vi "LogicEditor.vi"(1 "Logic Express":string) -> (0 "LogicExpressOut":string)   [LabVIEW 2020]
uses:
  <vilib>/Utility/miscctls.llb/LVPointTypeDef.ctl
panel:
  out "Operand2":string[](array[string])=[" ==NULL ", " ==EXIST ", " !=NULL ", " !=EXIST ", " ==[] ", " ==[;;] ", " !=[] ", " !=[;;] ", "@", " "]
  out "Operand":string[](array[string])=[" & ", " | ", "~", " ( ", " ) ", " == ", " != ", " >= ", " <= ", " > ", " < ", " <>", " </>", "~"]
  in  "Section":string(combo)
  out "VariableList":string[](array[string])
  out "IOList":string[](array[string])
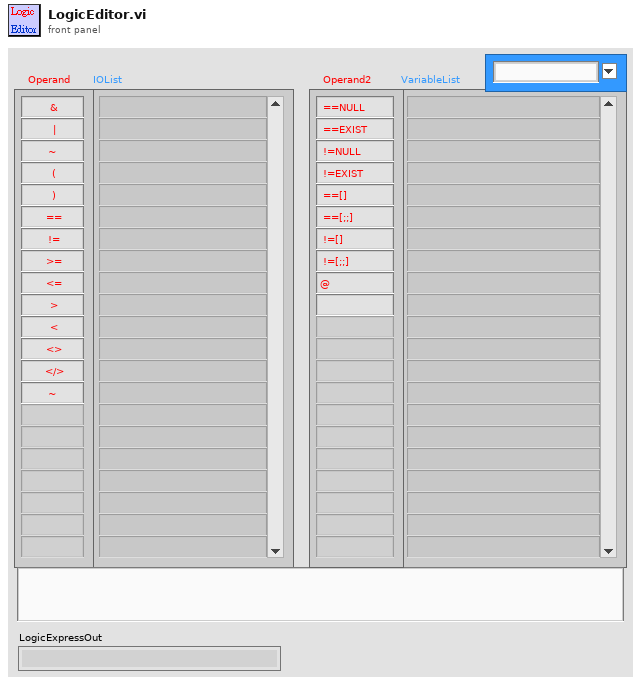
[diagram p1: front panel]
types:
  T1 = typedef "LVPointTypeDef.ctl" = cluster{"Horizontal":i16, "Vertical":i16}
  T2 = enum16{"Get", "Init", "Set", "Delete", "GetElement", "Inc", "Dec", "ReName"}
  T3 = typedef "LVPoint32TypeDef.ctl" = cluster{"Horizontal":i32, "Vertical":i32}
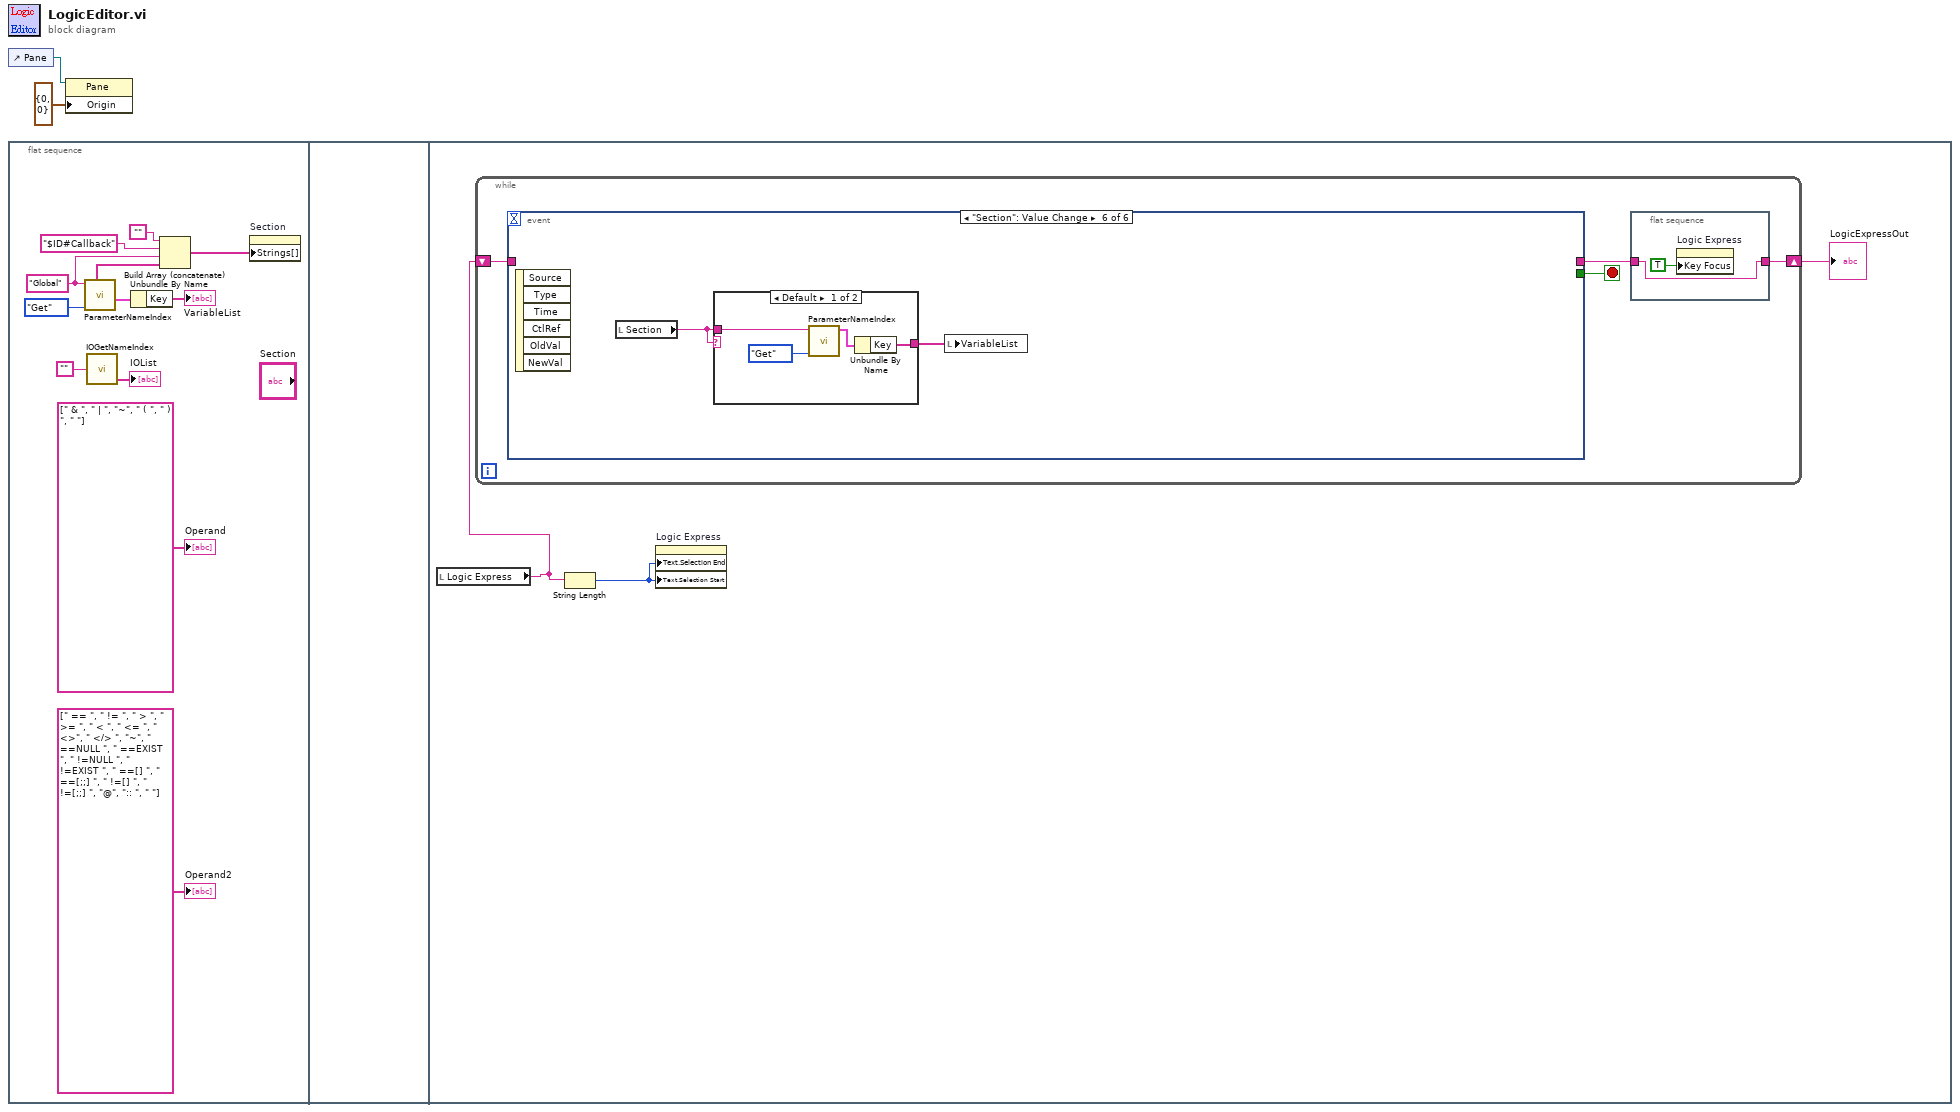
[diagram p0: block diagram]
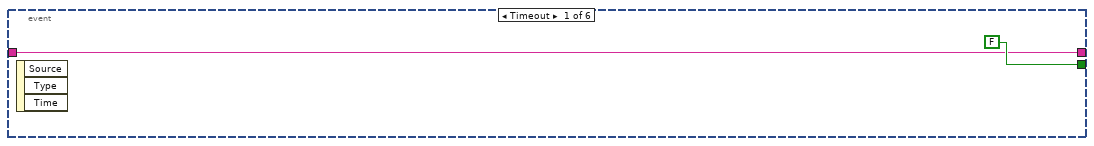
[diagram p2: hidden frame]
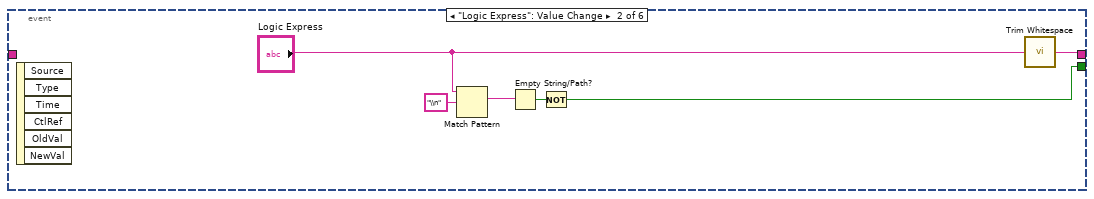
[diagram p3: hidden frame]
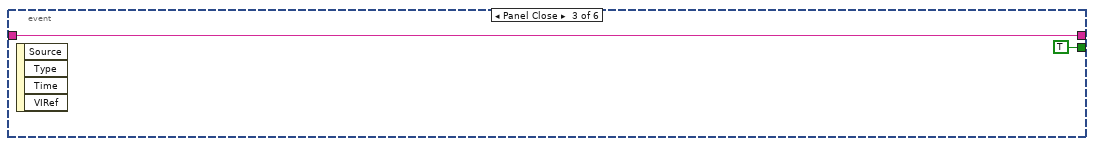
[diagram p4: hidden frame]
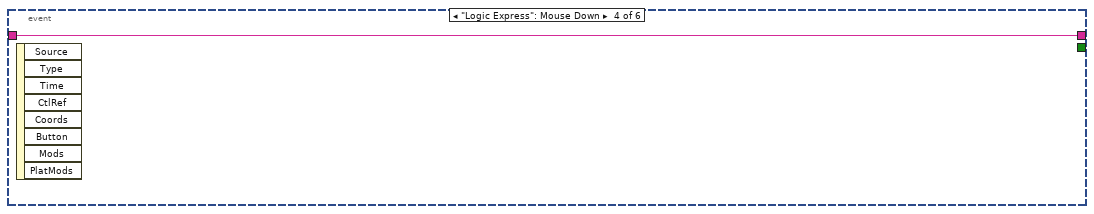
[diagram p5: hidden frame]
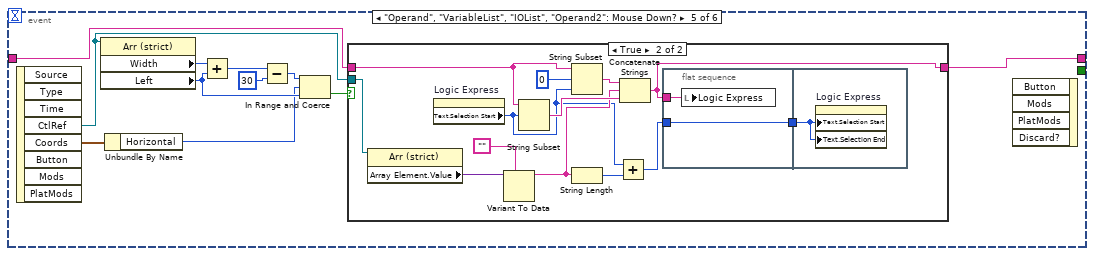
[diagram p6: hidden frame]
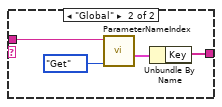
[diagram p8: hidden frame]
diagram:
  n1 = control-ref of="Pane"() -> (w2:refnum<vi>)
  n2 = flat-sequence {
    frame #0 {
      w7 = "Global" ("VariableSection")
      n3 = call "ParameterNameIndex.vi"("OP"=T2."Get", "VariableSection"=w7) -> ("GlobalKeyValue"=w11:cluster{"Key":string[], "Value":string[]}, "SectionList"=w6:string[])  [unwired: 3 in, 5 out]
      n4 = call "IOGetNameIndex.vi"("PortName"="") -> ("PortNameList Out"=→"IOList":string[])  [unwired: 3 in, 1 out]
      n5 = Unbundle By Name(w11) -> ("Key"=→"VariableList":string[])
      n6 = Build Array (concatenate)("", "$ID#Callback" ("VariableSection"), w7, w6) -> (w5:string[])
      n7 = property on="Section" class="CmbBox"("Strings[]"=w5) -> ()  [unwired: 2 in, 2 out]
      "Operand" <- string[] [" & ", " | ", "~", " ( ", " ) ", " "] ("Operate")
      "Operand2" <- string[] [" == ", " != ", " > ", " >= ", " < ", " <= ", " <>", " </> ", "~", " ==NULL ", " ==EXIST ", " !=NULL ", " !=EXIST ", " ==[] ", " ==[;;] ", " !=[] ", " !=[;;] ", "@", ":: ", " "] ("Operate")
    }
    frame #1 {
    }
    frame #2 {
      n8 = local read "Logic Express"() -> (w15:string)
      n9 = while {
        shift-right: [w18] -> w17
        shift-left: w15 -> [w20]
        stop <- w21 stop-if-true
        n10 = event shown="[5] \"Section\": Value Change" {
          selector: _ -> [_ _ _ _ _ _]
          dyn-events: _ -> [_ _ _ _ _ _]
          timeout: _ -> [_ _ _ _ _ _]
          tunnel: [FALSE w26 TRUE _ _ _] -> w21
          tunnel: w20 -> [w24 _ w32 w34 w45 _]
          tunnel: [w24 w31 w32 w34 w44 _] -> w19
          event Timeout {
            n11 = event-data() -> ()  [unwired: 1 in, 3 out]
          }
          event "Logic Express": Value Change {
            n12 = event-data() -> ()  [unwired: 1 in, 6 out]
            n13 = Match Pattern(string="Logic Express", regular expression="\\n") -> (match substring=w28:string)  [unwired: 1 in, 3 out]
            n14 = Empty String/Path?(string/path=w28) -> (empty?=w27:bool)
            n15 = Not(x=w27) -> (.not. x?=w26:bool)
            n16 = call <vilib>:"Trim Whitespace.vi"("string"="Logic Express") -> ("trimmed string"=w31:string)  [unwired: 1 in]
          }
          event Panel Close {
            n17 = event-data() -> ()  [unwired: 1 in, 4 out]
          }
          event "Logic Express": Mouse Down {
            n18 = event-data() -> ()  [unwired: 1 in, 8 out]
          }
          event "Operand", "VariableList", "IOList", "Operand2": Mouse Down? {
            n19 = event-data() -> ("CtlRef"=w43:refnum<vi>, "Coords"=w42:T3)  [unwired: 1 in, 6 out]
            n20 = property class="Arr (strict)"(reference=w43) -> ("Width"=w41:u32, "Left"=w40:i32)  [unwired: 1 in, 2 out]
            n21 = Unbundle By Name(w42) -> ("Horizontal"=w36:i32)
            n22 = Add(x=w41, y=w40) -> (x+y=w39:u32)
            n23 = Subtract(x=w39, y=u32 30) -> (x-y=w37:u32)
            n24 = In Range and Coerce(upper limit=w37, x=w36, lower limit=w40) -> (In Range?=w35:bool)  [unwired: 1 out]
            n25 = case shown="True" w35 {
              tunnel: w45 -> [w46 w55]
              tunnel: [w46 w52] -> w44
              tunnel: w43 -> [_ w47]
              frame False {
              }
              frame True {
                n26 = property class="Arr (strict)"(reference=w47) -> ("Array Element.Value"=w58:variant)  [unwired: 1 in, 2 out]
                n27 = property on="Logic Express" class="Str"() -> ("Text.Selection Start"=w49:u32)  [unwired: 2 in, 2 out]
                n28 = Variant To Data(type="", Variant=w58) -> (data=w51:string)  [unwired: 1 in, 1 out]
                n29 = String Subset(string=w55, offset (0)=w49) -> (substring=w53:string)  [unwired: 1 in]
                n30 = String Subset(string=w55, offset (0)=0, length (rest)=w49) -> (substring=w54:string)
                n31 = String Length(string=w51) -> (length=w50:i32)
                n32 = Add(x=w49, y=w50) -> (x+y=w48:u32)
                n33 = Concatenate Strings(w54, w51, w53) -> (w52:string)
                n34 = flat-sequence {
                  tunnel: w52 -> [w61]
                  tunnel: [w60] -> w59
                  tunnel: w48 -> [w60]
                  tunnel: w59 -> [w62]
                  frame #0 {
                    n35 = local write "Logic Express"(w61) -> ()
                  }
                  frame #1 {
                    n36 = property on="Logic Express" class="Str"("Text.Selection Start"=w62, "Text.Selection End"=w62) -> ()  [unwired: 2 in, 2 out]
                  }
                }
              }
            }
            n37 = event-data() -> ()  [unwired: 5 in, 1 out]
          }
          event "Section": Value Change {
            n38 = event-data() -> ()  [unwired: 1 in, 6 out]
            n39 = local read "Section"() -> (w63:string)
            n40 = case shown="Default" w63 {
              tunnel: [w65 w71] -> w64
              tunnel: w63 -> [w66 w70]
              frame Default {
                n41 = call "ParameterNameIndex.vi"("OP"=T2."Get", "VariableSection"=w66) -> ("SectionKeyValue"=w67:cluster{"Key":string[], "Value":string[]})  [unwired: 3 in, 6 out]
                n42 = Unbundle By Name(w67) -> ("Key"=w65:string[])
              }
              frame "Global" {
                n43 = call "ParameterNameIndex.vi"("OP"=T2."Get", "VariableSection"=w70) -> ("GlobalKeyValue"=w69:cluster{"Key":string[], "Value":string[]})  [unwired: 3 in, 6 out]
                n44 = Unbundle By Name(w69) -> ("Key"=w71:string[])
              }
            }
            n45 = local write "VariableList"(w64) -> ()
          }
        }
        n46 = flat-sequence {
          tunnel: w19 -> [w23]
          tunnel: [w23] -> w18
          frame #0 {
            n47 = property on="Logic Express" class="Str"("Key Focus"=TRUE) -> ()  [unwired: 2 in, 2 out]
          }
        }
      }
      "LogicExpressOut" <- w17
      n48 = String Length(string=w15) -> (length=w16:i32)
      n49 = property on="Logic Express" class="Str"("Text.Selection End"=w16, "Text.Selection Start"=w16) -> ()  [unwired: 2 in, 2 out]
    }
  }
  n50 = property class="Pane"(reference=w2, "Origin"=T1 {"Horizontal"=0, "Vertical"=0}) -> ()  [unwired: 1 in, 2 out]
